vi "getINIPath.vi"(8 "error in (no error)":errorcluster, 10 "DeviceType Name":string="name", 11 "Device Name":string="name") -> (0 "error out":errorcluster, 3 "reference trace path":string)   [LabVIEW 2020]
uses:
  <vilib>/Utility/config.llb/Read Key (String).vi
  <vilib>/Utility/config.llb/NI_LVConfig.lvlib
panel:
  out "Application:Directory Path":path
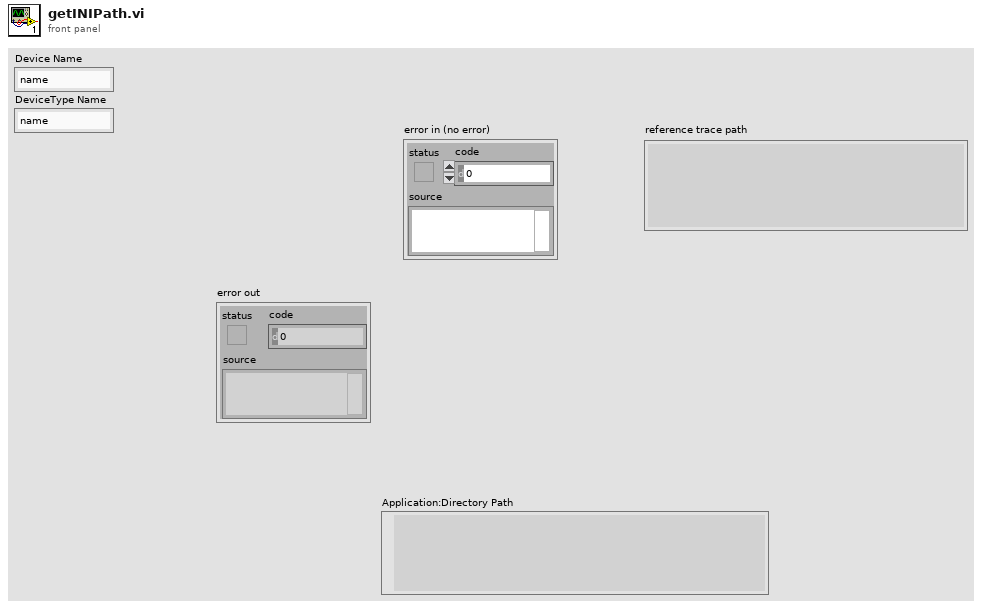
[diagram p1: front panel]
types:
  T1 = typedef "NI_LVConfig.lvlib/Config Data RefNum.ctl" = refnum<k1>
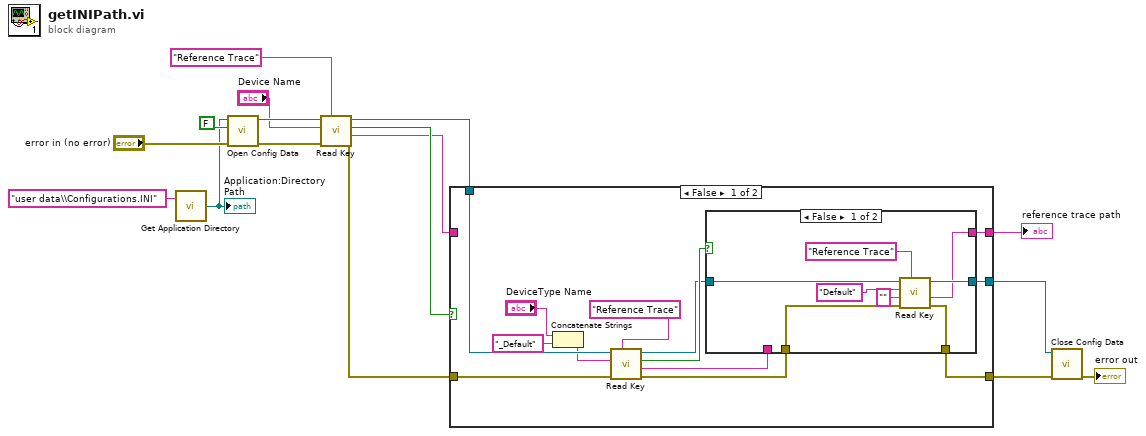
[diagram p0: block diagram]
diagram:
  n1 = call "Get Application Directory.vi"("name or relative path"="user data\\Configurations.INI") -> ("Path to config file"=w11:path)  [unwired: 1 in]
  "Application:Directory Path" <- w11
  n2 = call <vilib>:"Open Config Data.vi"("error in (no error)"="error in (no error)", "create file if necessary (T)"=FALSE, "configuration file path"=w11) -> ("error out"=w15:errorcluster, "refnum"=w13:T1)  [unwired: 6 in, 1 out]
  n3 = call-poly <vilib>:"Read Key.vi"("section"="Reference Trace", "error in (no error)"=w15, "key"="Device Name", "refnum"=w13) -> ("error out"=w4:errorcluster, "value"=w8:string, "found?"=w9:bool, "refnum out"=w5:T1)  [unwired: 4 in]
  n4 = case shown="False" w9 {
    tunnel: w8 -> [_ w43]
    tunnel: [w21 w43] -> w7
    tunnel: w5 -> [w28 w42]
    tunnel: w4 -> [w24 w41]
    tunnel: [w17 w41] -> w3
    tunnel: [w18 w42] -> w2
    frame False {
      n5 = Concatenate Strings("DeviceType Name", "_Default" ("string")) -> (w25:string)
      n6 = call-poly <vilib>:"Read Key.vi"("section"="Reference Trace", "error in (no error)"=w24, "key"=w25, "refnum"=w28) -> ("error out"=w20:errorcluster, "value"=w22:string, "found?"=w23:bool, "refnum out"=w19:T1)  [unwired: 4 in]
      n7 = case shown="False" w23 {
        tunnel: w22 -> [_ w40]
        tunnel: [w32 w40] -> w21
        tunnel: w20 -> [w35 w38]
        tunnel: w19 -> [w34 w39]
        tunnel: [w33 w39] -> w18
        tunnel: [w31 w38] -> w17
        frame False {
          n8 = call-poly <vilib>:"Read Key.vi"("section"="Reference Trace", "error in (no error)"=w35, "default value"="", "key"="Default" ("string"), "refnum"=w34) -> ("error out"=w31:errorcluster, "value"=w32:string, "refnum out"=w33:T1)  [unwired: 3 in, 1 out]
        }
        frame True {
        }
      }
    }
    frame True {
    }
  }
  "reference trace path" <- w7
  n9 = call <vilib>:"Close Config Data.vi"("error in (no error)"=w3, "refnum"=w2) -> ("error out"=→"error out":errorcluster)  [unwired: 8 in, 1 out]
